vi "Save to Excel - (3-17-10) (SubVI).vi"(0 "File Path Input":path, 1 "Save (Enable/Signal)":bool, 2 "Save Interval (s)":dbl=1.0, 3 "Title Block Array":string[](array[string]), 4 "Column Header Array":string[](array[string]), 5 "Data Array (Row)":string[](array[string]), 7 "File Configuration":T1={"Row Limit"=65500, "Default File Name"="Data", "New File Daily?"=TRUE, "Manual Save Interval?"=FALSE}, 9 "Change Save Location?":bool, 11 "Reset Elapsed Time":bool) -> (14 "File Path Output":path, 15 "Save Indicator":bool, 16 "# of Rows Saved":i32, 17 "Elapsed Time":string="00:00:00", 19 "Error Output":errorcluster)   [LabVIEW 2009]
panel:
  out "created path":path
  in  "Comments":string
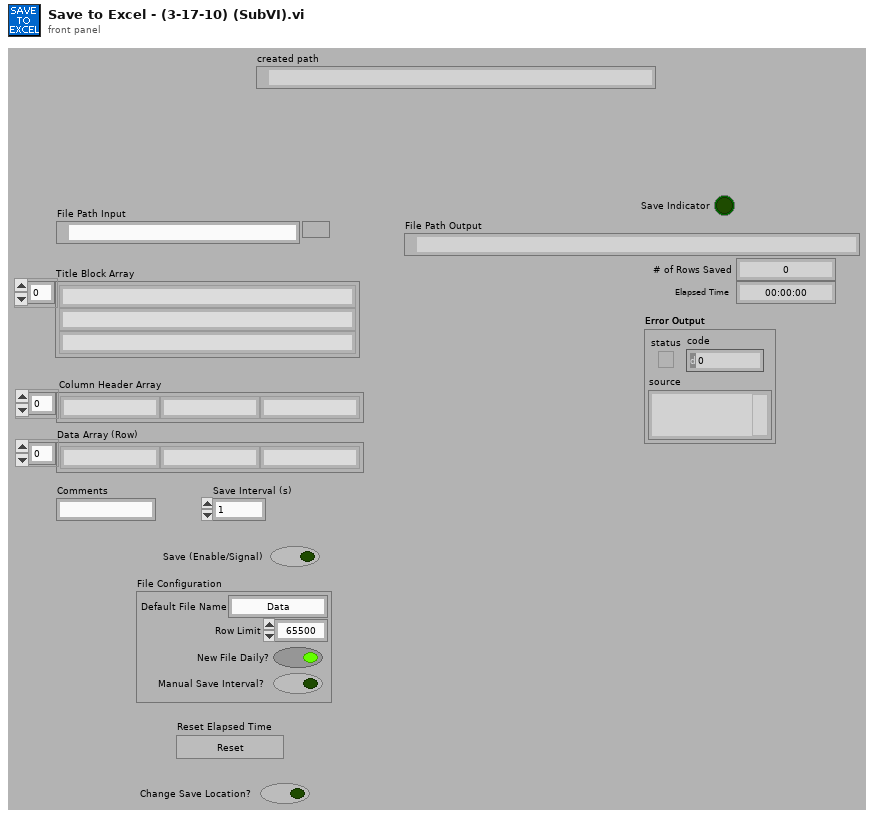
[diagram p1: front panel]
types:
  T1 = cluster{"Row Limit":i32, "Default File Name":string, "New File Daily?":bool, "Manual Save Interval?":bool}
  T2 = typedef "LVDateTimeRec.ctl" = cluster{"fractional second":dbl, "second":i32, "minute":i32, "hour":i32, "day of month":i32, "month":i32, "year":i32, "day of week":i32, "day of year":i32, "DST":i32}
  T3 = enum16{"open", "replace", "create", "open or create", "replace or create", "replace or create with confirmation"}
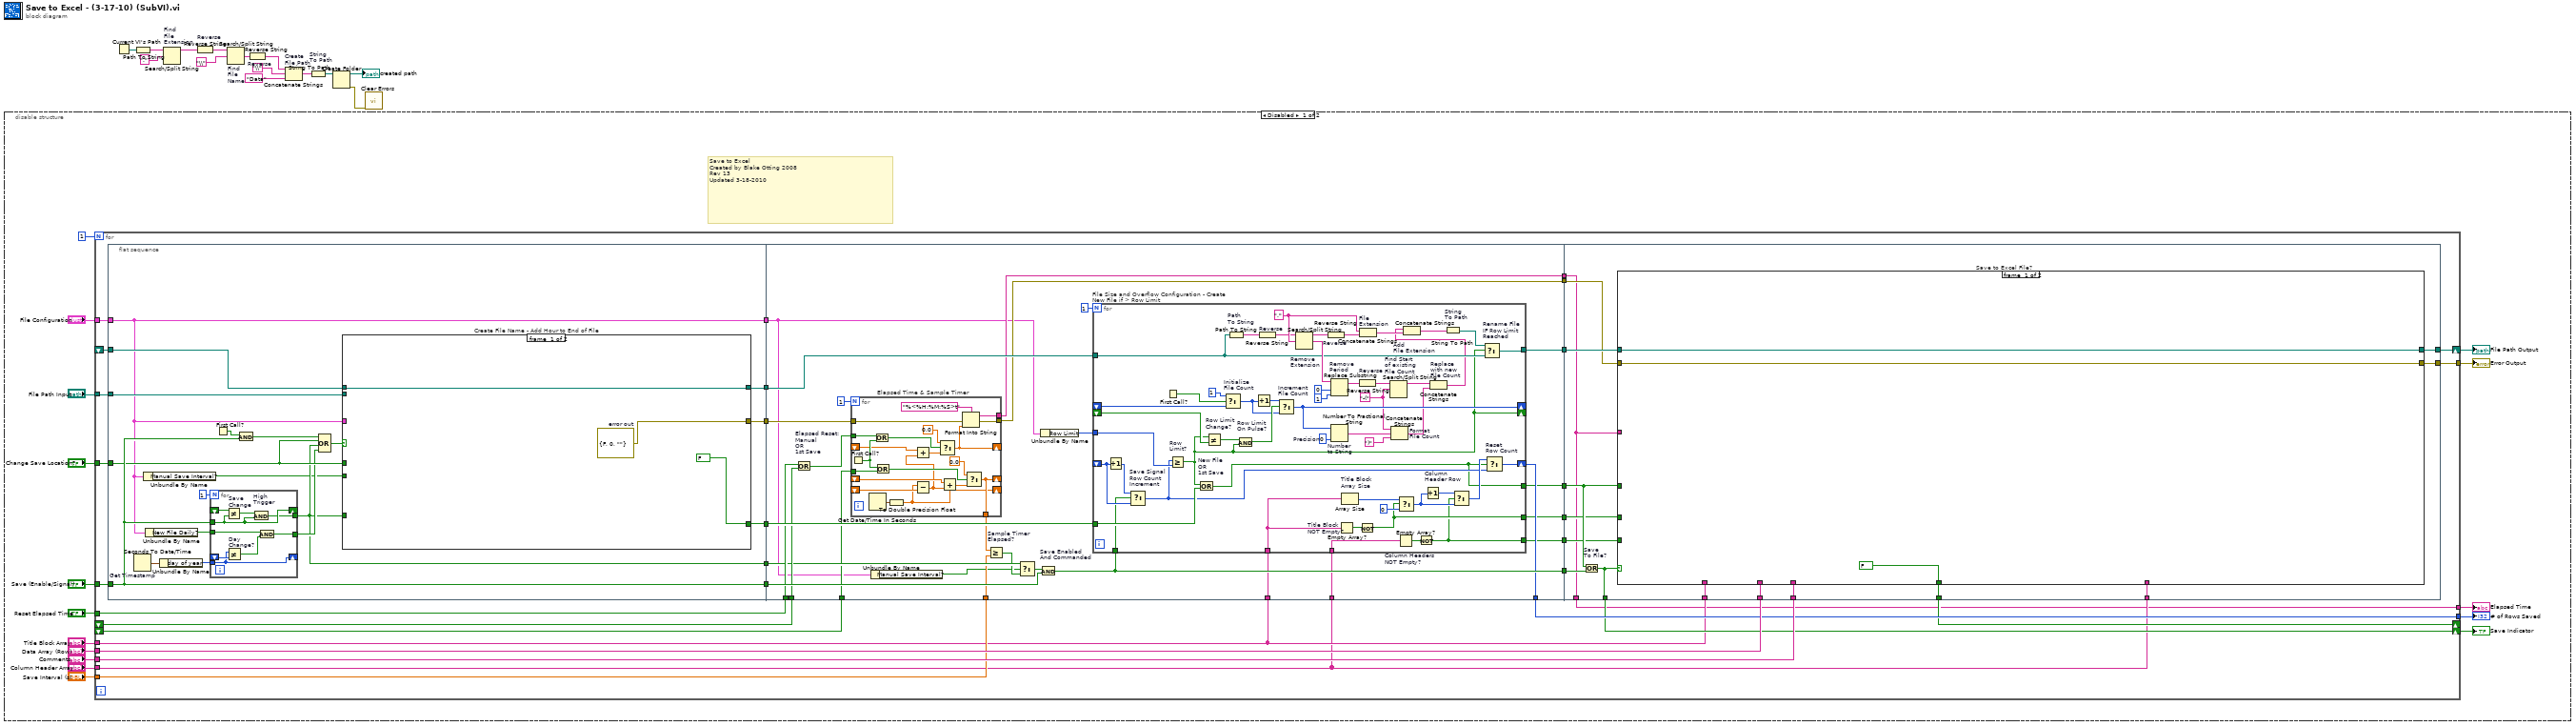
[diagram p0: block diagram]
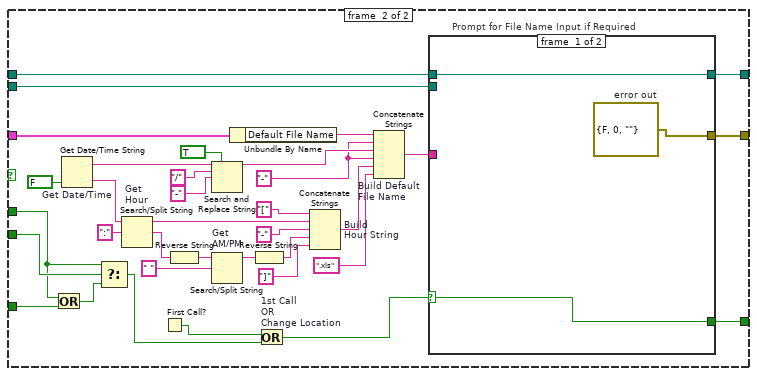
[diagram p2: hidden frame]
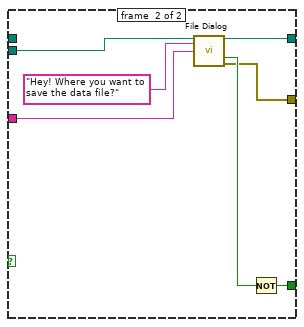
[diagram p3: hidden frame]
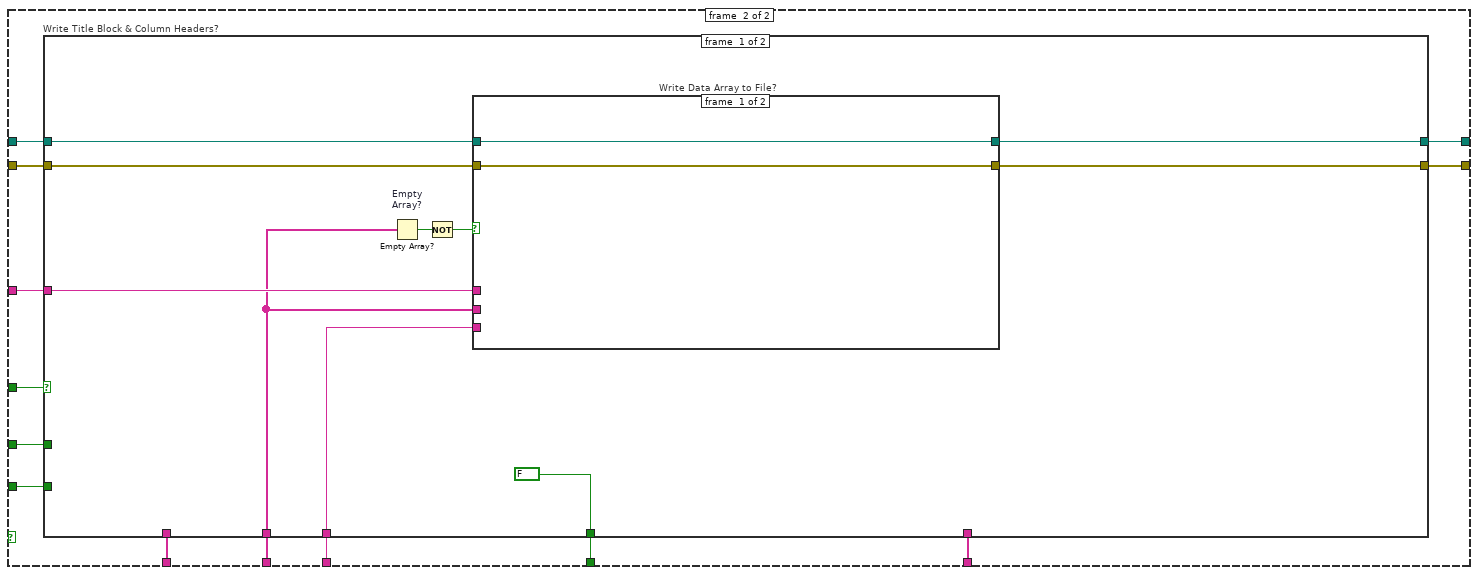
[diagram p4: hidden frame]
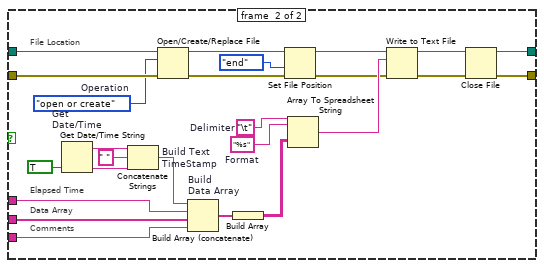
[diagram p5: hidden frame]
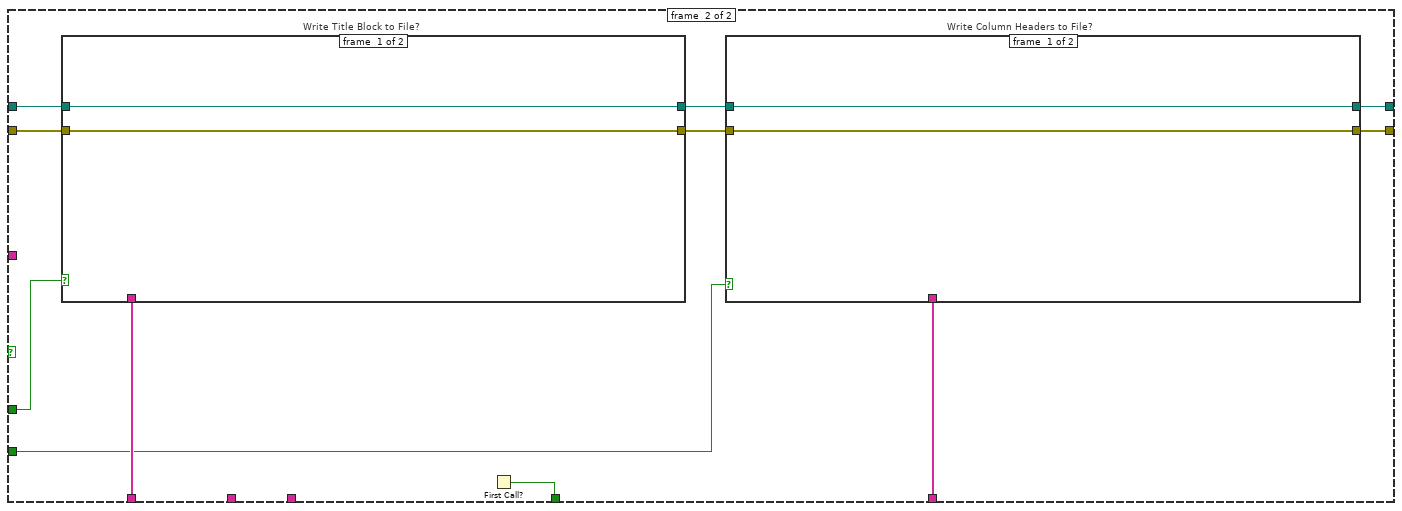
[diagram p6: hidden frame]
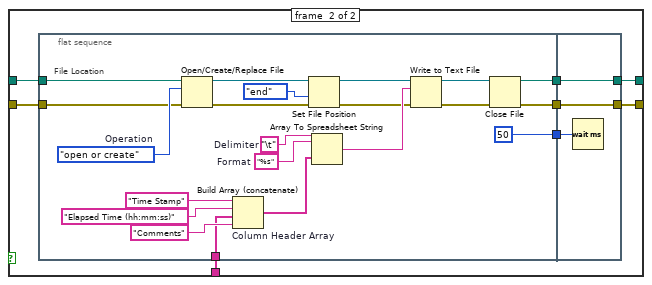
[diagram p7: hidden frame]
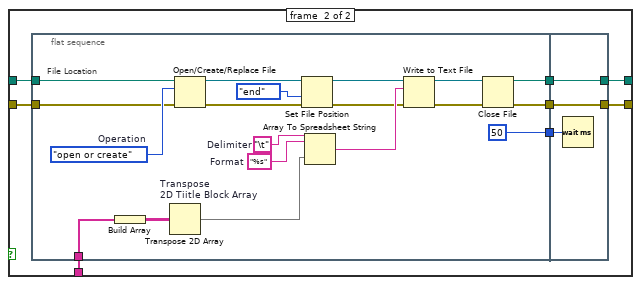
[diagram p8: hidden frame]
diagram:
  n1 = disable-structure shown="Disabled" {
    frame #0 {
      # "Save to Excel\nCreated by Blake Otting 2008\nRev 13\nUpdated 3-18-2010"
      n2 = for {
        N: 1 -> [_]
        tunnel: "File Path Input" -> [w52]
        tunnel: "Change Save Location?" -> [w62]
        tunnel: "Save (Enable/Signal)" -> [w46]
        tunnel: "Data Array (Row)" -> [w54]
        tunnel: "Column Header Array" -> [w36]
        tunnel: "File Configuration" -> [w42]
        tunnel: "Reset Elapsed Time" -> [w43]
        shift-right: [w48] -> w29
        shift-left: _ -> [w58]
        tunnel: "Save Interval (s)" -> [w47]
        shift-right: [w49] -> _
        shift-left: _ -> [w44]
        tunnel: "Title Block Array" -> [w38]
        tunnel: "Comments" -> [w53]
        shift-right: [w55] -> w27
        shift-left: _ -> [w51]
        tunnel: [w32] -> w28
        tunnel: [w50] -> w30
        tunnel: [w39] -> w15
        n3 = flat-sequence {
          tunnel: w51 -> [w78]
          tunnel: w52 -> [w77]
          tunnel: w62 -> [w68]
          tunnel: w42 -> [w64]
          tunnel: [w80] -> w61
          tunnel: [w79] -> w60
          tunnel: [w76] -> w59
          tunnel: w46 -> [w70]
          tunnel: [w70] -> w45
          tunnel: [w65] -> w41
          tunnel: [w64] -> w31
          tunnel: [w164] -> w57
          tunnel: [w141] -> w56
          tunnel: w58 -> [w146]
          tunnel: w59 -> [w154]
          tunnel: w60 -> [w144]
          tunnel: w61 -> [w165]
          tunnel: [w156] -> w50
          tunnel: w47 -> [w143]
          tunnel: w45 -> [w162]
          tunnel: w44 -> [w159]
          tunnel: w43 -> [w158]
          tunnel: w41 -> [w157]
          tunnel: [w147] -> w40
          tunnel: w38 -> [w155]
          tunnel: [w153] -> w37
          tunnel: w36 -> [w152]
          tunnel: [w151] -> w35
          tunnel: [w150] -> w34
          tunnel: [w140] -> w33
          tunnel: w31 -> [w139]
          tunnel: w57 -> [w252]
          tunnel: w56 -> [w238]
          tunnel: [w250] -> w55
          tunnel: w38 -> [w249]
          tunnel: w54 -> [w248]
          tunnel: w36 -> [w247]
          tunnel: w53 -> [w246]
          tunnel: [w245] -> w48
          tunnel: [w244] -> w49
          tunnel: w40 -> [w243]
          tunnel: [w242] -> w39
          tunnel: w37 -> [w251]
          tunnel: w35 -> [w241]
          tunnel: w34 -> [w240]
          tunnel: w33 -> [w239]
          tunnel: [w238] -> w32
          frame #0 {
            n4 = Seconds To Date/Time "Get Timestamp"() -> (date time rec=w73:T2)  [unwired: 2 out]
            n5 = Unbundle By Name(w64) -> ("Manual Save Interval?"=w63:bool)
            n6 = Unbundle By Name(w64) -> ("New File Daily?"=w75:bool)
            n7 = Unbundle By Name(w73) -> ("day of year"=w74:i32)
            n8 = for {
              N: 1 -> [_]
              tunnel: w70 -> [w87]
              shift-right: [w87] -> _
              shift-left: _ -> [w89]
              tunnel: [w86] -> w65
              tunnel: w74 -> [w84]
              shift-right: [w84] -> _
              shift-left: _ -> [w85]
              tunnel: w75 -> [w82]
              tunnel: [w81] -> w67
              n9 = Not Equal? "Save\nChange"(x=w89, y=w87) -> (x != y?=w88:bool)
              n10 = Not Equal? "Day\nChange?"(x=w84, y=w85) -> (x != y?=w83:bool)
              n11 = And "High\nTrigger"(x=w88, y=w87) -> (x .and. y?=w86:bool)
              n12 = And(x=w82, y=w83) -> (x .and. y?=w81:bool)
            }
            n13 = First Call?() -> (First Call?: T/F=w71:bool)
            n14 = And(x=w71, y=w70) -> (x .and. y?=w69:bool)
            n15 = Compound Arithmetic op=OR(w69, w68, w65, w67) -> (w66:bool)
            n16 = case "Create File Name - Add Hour to End of File" shown="True" w66 {
              tunnel: [w92 w124] -> w76
              tunnel: w78 -> [w92 w98]
              tunnel: [FALSE ("First Call?: T/F") w126] -> w80
              tunnel: w77 -> [_ w125]
              tunnel: w68 -> [_ w95]
              tunnel: [w90 w123] -> w79
              tunnel: w64 -> [_ w118]
              tunnel: w65 -> [_ w97]
              tunnel: w63 -> [_ w96]
              frame #0 {
                w90 = errorcluster {"status"=FALSE, "code"=0, "source"=""}  # error out
              }
              frame #1 {
                w108 = "-" ("string")
                n17 = Or(x=w95, y=w97) -> (x .or. y?=w94:bool)
                n18 = Get Date/Time String "Get Date/Time"(want seconds? (F)=FALSE) -> (date string=w102:string, time string=w101:string)  [unwired: 2 out]
                n19 = Select(t=w95, s=w96, f=w94) -> (s? t:f=w93:bool)
                n20 = Search/Split String "Get\nHour"(string=w101, search string/char (-)=":" ("search string")) -> (substring before match=w114:string, match + rest of string=w110:string)  [unwired: 2 out]
                n21 = First Call?() -> (First Call?: T/F=w99:bool)
                n22 = Reverse String(1:w110) -> (0:w111:string)
                n23 = Search and Replace String(replace all?=TRUE ("replace all? (F)"), input string=w102, search string="/", replace string="-" ("replace string (\"\")")) -> (result string=w121:string)  [unwired: 1 in, 6 out]
                n24 = Search/Split String "Get\nAM/PM"(string=w111, search string/char (-)=" ") -> (substring before match=w113:string)  [unwired: 3 out]
                n25 = Unbundle By Name(w118) -> ("Default File Name"=w122:string)
                n26 = Reverse String(1:w113) -> (0:w115:string)
                n27 = Or "1st Call\nOR\nChange Location"(x=w99, y=w93) -> (x .or. y?=w127:bool)
                n28 = Concatenate Strings "Build\nHour String"("[" ("string"), w114, "-" ("search string/char (-)"), w115, "]" ("string")) -> (w104:string)
                n29 = Concatenate Strings "Build Default\nFile Name"(w122, w108, w121, w108, w104, ".xls" ("string")) -> (w117:string)
                n30 = case "Prompt for File Name Input if Required" shown="True" w127 {
                  selector: w127 -> [w129 _]
                  tunnel: [w129 w136] -> w126
                  tunnel: w125 -> [_ w135]
                  tunnel: [w130 w134] -> w124
                  tunnel: w98 -> [w130 _]
                  tunnel: [w128 w132] -> w123
                  tunnel: w117 -> [_ w131]
                  frame #0 {
                    w128 = errorcluster {"status"=FALSE, "code"=0, "source"=""}  # error out
                  }
                  frame #1 {
                    n31 = call "File Dialog"("start path"=w135, "prompt"="Hey! Where you want to save the data file?", "default name"=w131) -> ("selected path"=w134:path, "cancelled"=w137:bool, "error out"=w132:errorcluster)  [unwired: 4 in, 6 out]
                    n32 = Not(x=w137) -> (.not. x?=w136:bool)
                  }
                }
              }
            }
          }
          frame #1 {
            n33 = Or "Elapsed Reset:\nManual\nOR\n1st Save"(x=w158, y=w159) -> (x .or. y?=w142:bool)
            n34 = for "Elapsed Time & Sample Timer" {
              N: 1 -> [_]
              shift-right: [w183] -> _
              shift-left: _ -> [w186]
              shift-right: [w175] -> _
              shift-left: _ -> [w185]
              tunnel: [w183] -> w148
              tunnel: w146 -> [w179]
              tunnel: w142 -> [w177]
              shift-right: [w170] -> _
              shift-left: _ -> [w174]
              tunnel: [w168] -> w141
              tunnel: [w167] -> w147
              tunnel: w144 -> [w166]
              n35 = First Call?() -> (First Call?: T/F=w178:bool)
              n36 = Get Date/Time In Seconds() -> (seconds since 1Jan1904=w184:timestamp)
              n37 = Or(x=w177, y=w178) -> (x .or. y?=w172:bool)
              n38 = Or(x=w178, y=w179) -> (x .or. y?=w180:bool)
              n39 = To Double Precision Float(number=w184) -> (double precision float=w175:dbl)
              n40 = Subtract(x=w175, y=w185) -> (x-y=w169:dbl)
              n41 = Add(x=w174, y=w169) -> (x+y=w176:dbl)
              n42 = Select(t=0.0, s=w172, f=w176) -> (s? t:f=w170:dbl)
              n43 = Add(x=w186, y=w169) -> (x+y=w182:dbl)
              n44 = Format Into String(format string="%<%H:%M:%S>t", error in=w166, w170) -> (resulting string=w168:string, error out=w167:errorcluster)  [unwired: 1 in]
              n45 = Select(t=0.0, s=w180, f=w182) -> (s? t:f=w183:dbl)
            }
            n46 = Unbundle By Name(w139) -> ("Manual Save Interval?"=w138:bool)
            n47 = Greater Or Equal? "Sample Timer\nElapsed?"(x=w148, y=w143) -> (x >= y?=w145:bool)
            n48 = Select(t=w157, s=w138, f=w145) -> (s? t:f=w163:bool)
            n49 = And "Save Enabled\nAnd Commanded"(x=w163, y=w162) -> (x .and. y?=w164:bool)
            n50 = Unbundle By Name(w139) -> ("Row Limit"=w161:i32)
            n51 = for "File Size and Overflow Configuration - Create New File if > Row Limit" {
              N: 1 -> [_]
              tunnel: w165 -> [w235]
              tunnel: w164 -> [w234]
              shift-right: [w232] -> w156
              shift-left: _ -> [w236]
              tunnel: w161 -> [w233]
              shift-right: [w200] -> _
              shift-left: _ -> [w231]
              tunnel: w155 -> [w196]
              shift-right: [w225] -> _
              shift-left: _ -> [w203]
              tunnel: w154 -> [w214]
              tunnel: [w206] -> w153
              tunnel: w152 -> [w198]
              tunnel: [w190] -> w150
              tunnel: [w189] -> w140
              tunnel: [w187] -> w151
              w223 = "." ("search string/char (-)")
              w207 = "-("
              w229 = i16 0  # Precision
              n52 = Increment(x=w236) -> (x+1=w237:i32)
              n53 = Select "Save Signal\nRow Count\nIncrement"(t=w237, s=w234, f=w236) -> (s? t:f=w188:i32)
              n54 = First Call?() -> (First Call?: T/F=w204:bool)
              n55 = Greater Or Equal? "Row\nLimit?"(x=w188, y=w233) -> (x >= y?=w200:bool)
              n56 = Or "New File\nOR\n1st Save"(x=w200, y=w235) -> (x .or. y?=w187:bool)
              n57 = Not Equal? "Row Limit\nChange?"(x=w200, y=w231) -> (x != y?=w226:bool)
              n58 = Select "Initialize\nFile Count"(t=i16 1, s=w204, f=w203) -> (s? t:f=w202:i16)
              n59 = Path To String "Path\nTo String"(path=w214) -> (string=w216:string)
              n60 = And "Row Limit\nOn Pulse?"(x=w226, y=w200) -> (x .and. y?=w230:bool)
              n61 = Increment(x=w202) -> (x+1=w227:i16)
              n62 = Reverse String "Reverse"(1:w216) -> (0:w217:string)
              n63 = Select "Increment\nFile Count"(t=w227, s=w230, f=w202) -> (s? t:f=w225:i16)
              n64 = Search/Split String "Remove\nExtension"(string=w217, search string/char (-)=w223) -> (substring before match=w218:string, match + rest of string=w219:string)  [unwired: 2 out]
              n65 = Reverse String "Reverse"(1:w218) -> (0:w215:string)
              n66 = Replace Substring "Remove\nPeriod"(2:1 ("length (len. of substring)"), 3:0 ("offset (0)"), 5:w219) -> (1:w220:string)  [unwired: 2 out]
              n67 = Number To Fractional String "Number\nto String"(number=w225, precision (6)=w229) -> (F-format string=w228:string)  [unwired: 2 in]
              n68 = Empty Array? "Title Block\nNOT Empty?"(array=w196) -> (empty?=w197:bool)
              n69 = Array Size "Title Block\nArray Size"(array=w196) -> (size(s)=w195:i32)
              n70 = Reverse String "Reverse"(1:w220) -> (0:w212:string)
              n71 = Not(x=w197) -> (.not. x?=w190:bool)
              n72 = Concatenate Strings "File\nExtension"(w223, w215) -> (w209:string)
              n73 = Search/Split String "Find Start\nof existing\nFile Count"(string=w212, search string/char (-)=w207) -> (substring before match=w211:string)  [unwired: 1 in, 2 out]
              n74 = Concatenate Strings "Format\nFile Count"(w207, w228, ")") -> (w210:string)
              n75 = Empty Array? "Column Headers\nNOT Empty?"(array=w198) -> (empty?=w199:bool)
              n76 = Select(t=w195, s=w190, f=0 ("t")) -> (s? t:f=w193:i32)
              n77 = Not(x=w199) -> (.not. x?=w189:bool)
              n78 = Increment "Column\nHeader Row"(x=w193) -> (x+1=w192:i32)
              n79 = Concatenate Strings "Replace\nwith new\nFile Count"(w211, w210) -> (w201:string)
              n80 = Concatenate Strings "Add\nFile Extension"(w201, w209) -> (w208:string)
              n81 = String To Path "String\nTo Path"(string=w208) -> (path=w224:path)
              n82 = Select(t=w192, s=w189, f=w193) -> (s? t:f=w191:i32)
              n83 = Select "Rename File\nIF Row Limit\nReached"(t=w224, s=w200, f=w214) -> (s? t:f=w206:path)
              n84 = Select "Reset\nRow Count"(t=w191, s=w187, f=w188) -> (s? t:f=w232:i32)
            }
          }
          frame #2 {
            n85 = Or "Save\nTo File?"(x=w241, y=w252) -> (x .or. y?=w245:bool)
            n86 = case "Save to Excel File?" shown="True" w245 {
              tunnel: [w255 w268] -> w250
              tunnel: w251 -> [w255 w267]
              tunnel: w241 -> [_ w266]
              tunnel: [FALSE ("First Call?: T/F") w265] -> w244
              tunnel: w238 -> [_ w264]
              tunnel: w249 -> [_ w261]
              tunnel: w248 -> [_ w263]
              tunnel: w247 -> [_ w262]
              tunnel: w246 -> [_ w260]
              tunnel: w243 -> [w253 w259]
              tunnel: [w253 w258] -> w242
              tunnel: w240 -> [_ w257]
              tunnel: w239 -> [_ w256]
              frame #0 {
              }
              frame #1 {
                n87 = case "Write Title Block & Column Headers?" shown="True" w266 {
                  tunnel: [w276 w311] -> w268
                  tunnel: w267 -> [w277 w315]
                  tunnel: w261 -> [_ w309]
                  tunnel: w262 -> [_ w308]
                  tunnel: w264 -> [w275 _]
                  tunnel: [FALSE ("First Call?: T/F") w316] -> w265
                  tunnel: w260 -> [w273 _]
                  tunnel: w263 -> [w270 _]
                  tunnel: w259 -> [w274 w312]
                  tunnel: [w272 w310] -> w258
                  tunnel: w257 -> [_ w307]
                  tunnel: w256 -> [_ w306]
                  frame #0 {
                    n88 = Empty Array? "Empty\nArray?"(array=w270) -> (empty?=w271:bool)
                    n89 = Not(x=w271) -> (.not. x?=w269:bool)
                    n90 = case "Write Data Array to File?" shown="True" w269 {
                      tunnel: w277 -> [w280 w305]
                      tunnel: [w280 w304] -> w276
                      tunnel: w270 -> [_ w303]
                      tunnel: w275 -> [_ w302]
                      tunnel: w274 -> [w279 w301]
                      tunnel: w273 -> [_ w300]
                      tunnel: [w279 w299] -> w272
                      frame #0 {
                      }
                      frame #1 {
                        w288 = "\t"  # Delimiter
                        w287 = "%s"  # Format
                        w295 = T3."open or create"  # Operation
                        # "Comments"
                        # "Data Array"
                        # "Elapsed Time"
                        # "File Location"
                        n91 = Get Date/Time String "Get \nDate/Time"(want seconds? (F)=TRUE) -> (date string=w290:string, time string=w293:string)  [unwired: 2 out]
                        n92 = Concatenate Strings "Build Text\nTimeStamp"(w290, " " ("string"), w293) -> (w294:string)
                        n93 = Open/Create/Replace File(file path (use dialog)=w305, error in=w301, operation (0:open)=w295) -> (refnum out=w281:refnum<file>, error out=w282:errorcluster)  [unwired: 3 in, 1 out]
                        n94 = Build Array (concatenate) "Build\nData Array"(w294, w302, w303, w300) -> (w297:string[])
                        n95 = Build Array(w297) -> (w298:string[][])
                        n96 = Set File Position(refnum=w281, from (0:start)=enum16{"start", "end", "current"}."end", error in=w282) -> (refnum out=w283:refnum<file>, error out=w284:errorcluster)  [unwired: 1 in]
                        n97 = Array To Spreadsheet String(delimiter (Tab)=w288, array=w298, 3:w287) -> (spreadsheet string=w289:string)
                        n98 = Write to Text File(file (use dialog)=w283, text=w289, error in=w284) -> (refnum out=w285:refnum<file>, error out=w286:errorcluster)  [unwired: 1 in, 1 out]
                        n99 = Close File(refnum=w285, error in=w286) -> (path=w304:path, error out=w299:errorcluster)
                      }
                    }
                  }
                  frame #1 {
                    n100 = case "Write Title Block to File?" shown="True" w307 {
                      tunnel: w315 -> [w351 w360]
                      tunnel: w309 -> [_ w359]
                      tunnel: [w352 w358] -> w313
                      tunnel: [w351 w357] -> w314
                      tunnel: w312 -> [w352 w356]
                      frame #0 {
                      }
                      frame #1 {
                        n101 = flat-sequence "Write to Excel File" {
                          tunnel: w359 -> [w363]
                          tunnel: w360 -> [w368]
                          tunnel: w356 -> [w362]
                          tunnel: [w367] -> w355
                          tunnel: [w366] -> w354
                          tunnel: [u32 50 ("milliseconds to wait")] -> w353
                          tunnel: [w381] -> w358
                          tunnel: [w382] -> w357
                          tunnel: w355 -> [w382]
                          tunnel: w354 -> [w381]
                          tunnel: w353 -> [w380]
                          frame #0 {
                            w376 = "\t"  # Delimiter
                            w375 = "%s"  # Format
                            w378 = T3."open or create"  # Operation
                            # "File Location"
                            n102 = Build Array(w363) -> (w365:string[][])
                            n103 = Transpose 2D Array "Transpose\n2D Tiitle Block Array"(2D array=w365) -> (transposed array=w364:string[][])
                            n104 = Open/Create/Replace File(file path (use dialog)=w368, error in=w362, operation (0:open)=w378) -> (refnum out=w369:refnum<file>, error out=w370:errorcluster)  [unwired: 3 in, 1 out]
                            n105 = Set File Position(refnum=w369, from (0:start)=enum16{"start", "end", "current"}."end", error in=w370) -> (refnum out=w371:refnum<file>, error out=w372:errorcluster)  [unwired: 1 in]
                            n106 = Array To Spreadsheet String(delimiter (Tab)=w376, array=w364, 3:w375) -> (spreadsheet string=w377:string)
                            n107 = Write to Text File(file (use dialog)=w371, text=w377, error in=w372) -> (refnum out=w373:refnum<file>, error out=w374:errorcluster)  [unwired: 1 in, 1 out]
                            n108 = Close File(refnum=w373, error in=w374) -> (path=w367:path, error out=w366:errorcluster)
                          }
                          frame #1 {
                            n109 = Wait (ms)(milliseconds to wait=w380) -> ()  [unwired: 1 out]
                          }
                        }
                      }
                    }
                    n110 = First Call?() -> (First Call?: T/F=w316:bool)
                    n111 = case "Write Column Headers to File?" shown="True" w306 {
                      tunnel: w314 -> [w317 w326]
                      tunnel: [w318 w325] -> w310
                      tunnel: w313 -> [w318 w324]
                      tunnel: [w317 w323] -> w311
                      tunnel: w308 -> [_ w322]
                      frame #0 {
                      }
                      frame #1 {
                        n112 = flat-sequence "Write to Excel File" {
                          tunnel: w326 -> [w336]
                          tunnel: w324 -> [w333]
                          tunnel: w322 -> [w328]
                          tunnel: [w335] -> w321
                          tunnel: [w334] -> w320
                          tunnel: [u32 50 ("milliseconds to wait")] -> w319
                          tunnel: [w349] -> w325
                          tunnel: [w350] -> w323
                          tunnel: w321 -> [w350]
                          tunnel: w320 -> [w349]
                          tunnel: w319 -> [w348]
                          frame #0 {
                            w344 = "\t"  # Delimiter
                            w343 = "%s"  # Format
                            w346 = T3."open or create"  # Operation
                            # "File Location"
                            n113 = Open/Create/Replace File(file path (use dialog)=w336, error in=w333, operation (0:open)=w346) -> (refnum out=w337:refnum<file>, error out=w338:errorcluster)  [unwired: 3 in, 1 out]
                            n114 = Build Array (concatenate) "Column Header Array"("Time Stamp", "Elapsed Time (hh:mm:ss)", w328, "Comments") -> (w329:string[])
                            n115 = Set File Position(refnum=w337, from (0:start)=enum16{"start", "end", "current"}."end", error in=w338) -> (refnum out=w339:refnum<file>, error out=w340:errorcluster)  [unwired: 1 in]
                            n116 = Array To Spreadsheet String(delimiter (Tab)=w344, array=w329, 3:w343) -> (spreadsheet string=w345:string)
                            n117 = Write to Text File(file (use dialog)=w339, text=w345, error in=w340) -> (refnum out=w341:refnum<file>, error out=w342:errorcluster)  [unwired: 1 in, 1 out]
                            n118 = Close File(refnum=w341, error in=w342) -> (path=w335:path, error out=w334:errorcluster)
                          }
                          frame #1 {
                            n119 = Wait (ms)(milliseconds to wait=w348) -> ()  [unwired: 1 out]
                          }
                        }
                      }
                    }
                  }
                }
              }
            }
          }
        }
      }
      "# of Rows Saved" <- w30
      "Save Indicator" <- w29
      "File Path Output" <- w27
      "Error Output" <- w15
      "Elapsed Time" <- w28
    }
    frame #1 {
    }
  }
  n120 = Current VI's Path() -> (path=w5:path)
  n121 = Path To String(path=w5) -> (string=w11:string)
  n122 = Search/Split String "Find\nFile \nExtension"(string=w11, search string/char (-)=".") -> (substring before match=w10:string)  [unwired: 1 in, 2 out]
  n123 = Reverse String "Reverse"(1:w10) -> (0:w9:string)
  n124 = Search/Split String "Find\nFile \nName"(string=w9, search string/char (-)="\\") -> (match + rest of string=w7:string)  [unwired: 1 in, 2 out]
  n125 = Reverse String "Reverse"(1:w7) -> (0:w6:string)
  n126 = Concatenate Strings "Create\nFile Path"(w6, "\\", "Data") -> (w13:string)
  n127 = String To Path "String\nTo Path"(string=w13) -> (path=w2:path)
  n128 = Create Folder(path (use dialog)=w2) -> (created path=→"created path":path, error out=w1:errorcluster)  [unwired: 2 in, 1 out]
  n129 = call <vilib>:"Clear Errors.vi"("error in (no error)"=w1) -> ()  [unwired: 6 in, 1 out]
